vi "Destroy.vi"(0 "reference in":refnum<class "Client.lvclass">, 11 "Error In":errorcluster) -> (4 "reference out":refnum<class "Client.lvclass">, 15 "Error Out":errorcluster)   [LabVIEW 2024, in "Client.lvclass"]
uses:
  Client.lvclass
  Client.lvclass/Client.ctl
  Receiver/MediaPlayer_class/MediaPlayer.lvclass
  Invoker/RemoteControl_class/RemoteControl.lvclass
panel:
  # "Connector Pane"
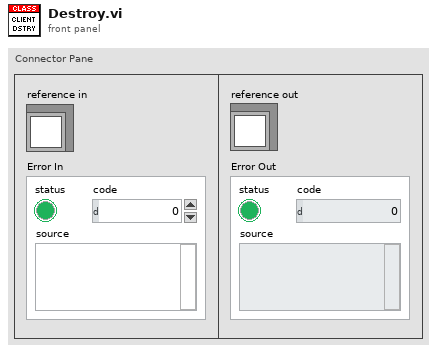
[diagram p1: front panel]
types:
  T1 = typedef "Client.lvclass/ObjectAttributes.ctl" = cluster{"RemoteControlRef":refnum<class "RemoteControl.lvclass">, "MediaPlayerRef":refnum<class "MediaPlayer.lvclass">, "Commands":cluster{"Play Music Command":refnum<class "IPlayerCommand.lvclass">, "Pause Music Command":refnum<class "IPlayerCommand.lvclass">, "Stop Music Command":refnum<class "IPlayerCommand.lvclass">, "Skip Music Command":refnum<class "IPlayerCommand.lvclass">, "Get Current Info Command":refnum<class "IPlayerCommand.lvclass">, "Rewind Music Command":refnum<class "IPlayerCommand.lvclass">}}
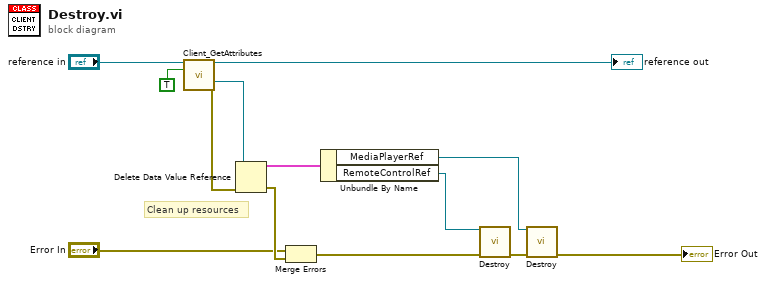
[diagram p0: block diagram]
diagram:
  # "Clean up resources"
  n1 = call "Client_GetAttributes.vi"("reference in"="reference in", "OnlyGetDvrReference(False)"=TRUE) -> ("reference out"=→"reference out":refnum<class "Client.lvclass">, "DataRef"=w11:refnum<data-value>, "Error Out"=w12:errorcluster)  [unwired: 10 in, 1 out]
  n2 = Delete Data Value Reference(data value reference=w11, error in=w12) -> (data value=w6:T1, error out=w10:errorcluster)
  n3 = Merge Errors("Error In", w10) -> (w2:errorcluster)
  n4 = Unbundle By Name(w6) -> ("MediaPlayerRef"=w3:refnum<class "MediaPlayer.lvclass">, "RemoteControlRef"=w5:refnum<class "RemoteControl.lvclass">)
  n5 = call-dynamic "Destroy.vi"("reference in"=w5, "Error In"=w2) -> ("Error Out"=w4:errorcluster)  [unwired: 12 in, 1 out]
  n6 = call-dynamic "Destroy.vi"("reference in"=w3, "Error In"=w4) -> ("Error Out"=→"Error Out":errorcluster)  [unwired: 12 in, 1 out]
